vi "Dialog3Stages.vi"(0 "X axis":T2={"Serial port handle"="", "Axis"="", "Controller #"=0, "Min position"=0.0, "Max position"=0.0, "Min velocity"=0.0, "Max velocity"=0.0, "Firmware"="", "Device ID"=0, "Variable event"=refnum, "Variable ref"=refnum, "Resolution, usteps/step"=0, "Serial port semaphore"=refnum, "Joystick buttons"={"MinDir"=1, "MaxDir"=2, "MedSpeed"=5, "HighSpeed"=6}} {"Joystick buttons"."HighSpeed" min=1 max=25 step=1; "Joystick buttons"."MedSpeed" min=1 max=25 step=1; "Joystick buttons"."MaxDir" min=1 max=25 step=1; "Joystick buttons"."MinDir" min=1 max=25 step=1}, 1 "Y axis":T2={"Serial port handle"="", "Axis"="", "Controller #"=0, "Min position"=0.0, "Max position"=0.0, "Min velocity"=0.0, "Max velocity"=0.0, "Firmware"="", "Device ID"=0, "Variable event"=refnum, "Variable ref"=refnum, "Resolution, usteps/step"=0, "Serial port semaphore"=refnum, "Joystick buttons"={"MinDir"=1, "MaxDir"=2, "MedSpeed"=5, "HighSpeed"=6}} {"Joystick buttons"."HighSpeed" min=1 max=25 step=1; "Joystick buttons"."MedSpeed" min=1 max=25 step=1; "Joystick buttons"."MaxDir" min=1 max=25 step=1; "Joystick buttons"."MinDir" min=1 max=25 step=1}, 2 "Z axis":T2={"Serial port handle"="", "Axis"="", "Controller #"=0, "Min position"=0.0, "Max position"=0.0, "Min velocity"=0.0, "Max velocity"=0.0, "Firmware"="", "Device ID"=0, "Variable event"=refnum, "Variable ref"=refnum, "Resolution, usteps/step"=0, "Serial port semaphore"=refnum, "Joystick buttons"={"MinDir"=1, "MaxDir"=2, "MedSpeed"=5, "HighSpeed"=6}} {"Joystick buttons"."HighSpeed" min=1 max=25 step=1; "Joystick buttons"."MedSpeed" min=1 max=25 step=1; "Joystick buttons"."MaxDir" min=1 max=25 step=1; "Joystick buttons"."MinDir" min=1 max=25 step=1}, 3 "Stop event":refnum<user-event>, 4 "Joystick event":T1, 5 "error in":errorcluster={"status"=FALSE, "code"=1073676294, "source"="VISA Read in Zaber TLCM.lvclass:Command.vi:1820008->Zaber TLCM.lvclass:Get home position.vi->Zaber TLCM.lvclass:Get limits.vi->Zaber TLCM.lvclass:Join.vi->Swan probe.vi"}) -> (19 "error out":errorcluster)   [LabVIEW 2018]
uses:
  Zaber.ctl
  GenericDataEvent/GenericEvent.ctl
  ZaberVariables.ctl
  Joystick events/Joystick event.ctl
  <vilib>/Analysis/baseanly.llb/Real Outer Product.vi
  <vilib>/Analysis/NI_AALBase.lvlib
panel:
  in  "ZSlide":dbl(slide)=38.4141345 caption="Z axis, mm" scale format="%#_3f"
  out "XYPositionGraph":dbl[][](graph) caption="XY position graph"
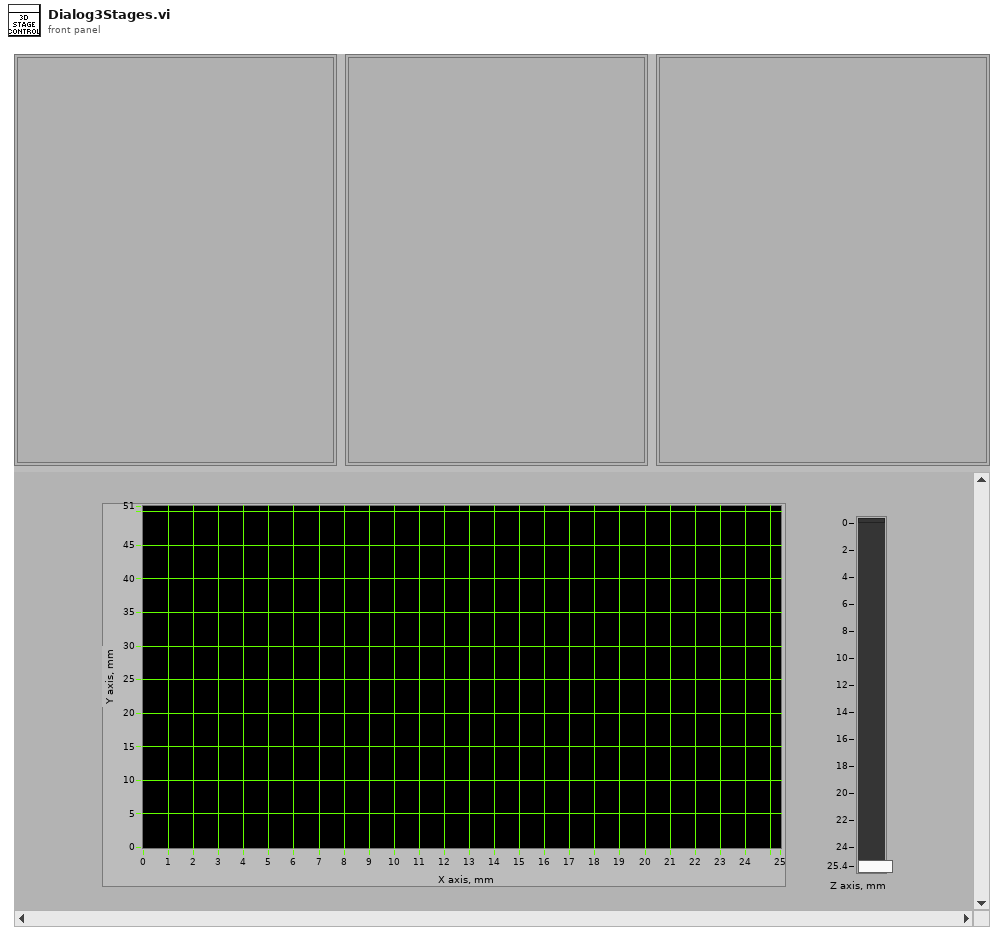
[diagram p1: front panel]
types:
  T1 = typedef "Joystick event.ctl" = refnum<user-event>
  T2 = typedef "Zaber.ctl" = cluster{"Serial port handle":refnum<visa-resource-name>, "Axis":string, "Controller #":u8, "Min position":dbl, "Max position":dbl, "Min velocity":dbl, "Max velocity":dbl, "Firmware":string, "Device ID":i32, "Variable event":T3, "Variable ref":refnum<data-value>, "Resolution, usteps/step":i32, "Serial port semaphore":T4, "Joystick buttons":cluster{"MinDir":i32, "MaxDir":i32, "MedSpeed":i32, "HighSpeed":i32}}
  T3 = typedef "GenericEvent.ctl" = refnum<user-event>
  T4 = typedef "Semaphore RefNum" = refnum<k1>
  T5 = typedef "NI_Matrix.lvlib/RealMatrix.ctl" = dbl[][]
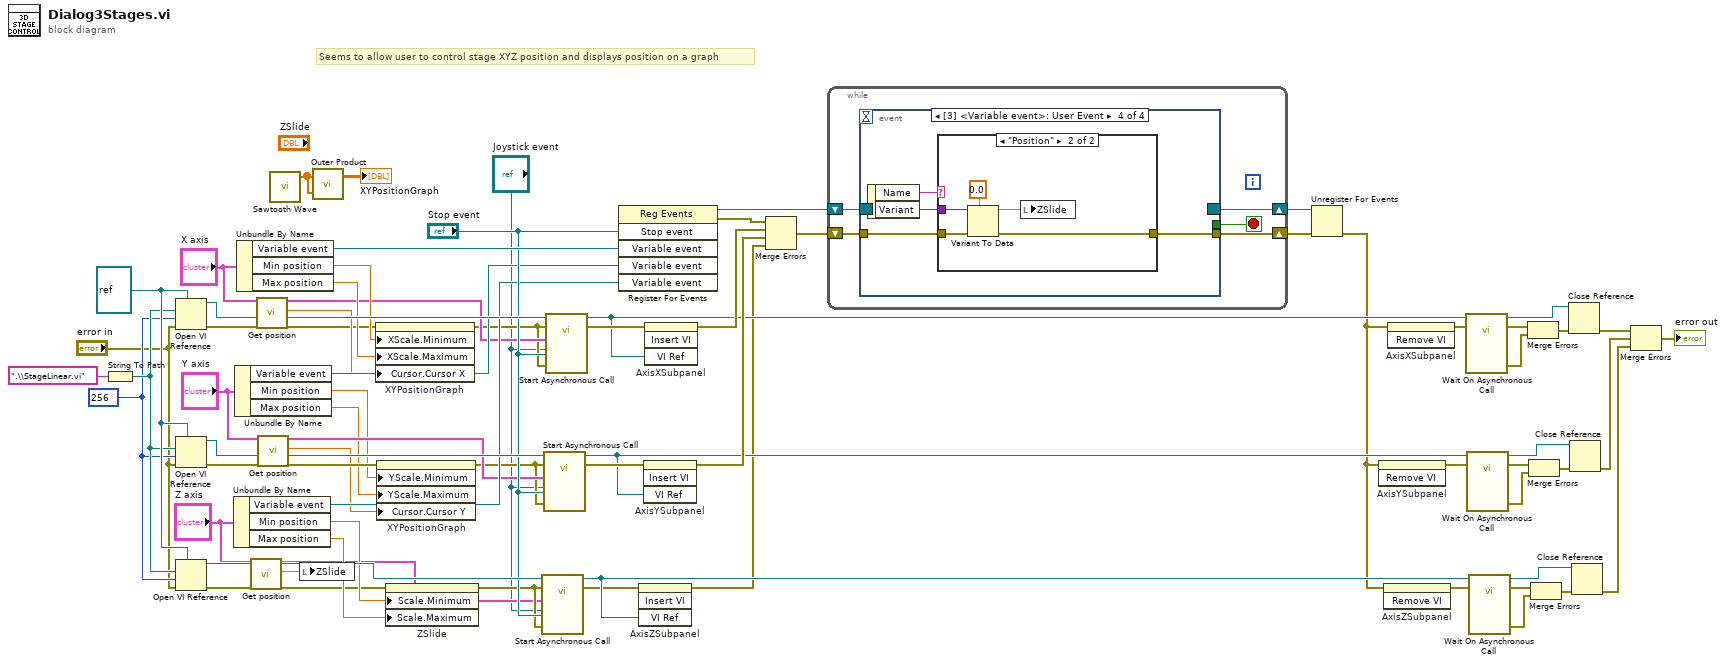
[diagram p0: block diagram]
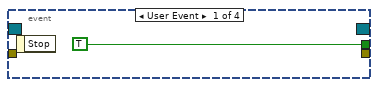
[diagram p2: hidden frame]
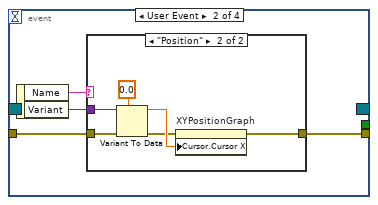
[diagram p3: hidden frame]
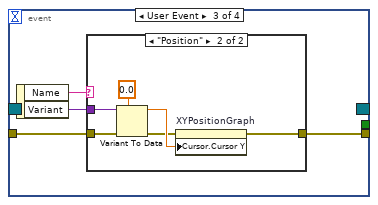
[diagram p5: hidden frame]
diagram:
  w62 = refnum<vi> refnum ("type specifier VI Refnum (for type only)")
  w60 = 256 ("options")
  # "Seems to allow user to control stage XYZ position and displays position on a graph"
  n1 = String To Path(string=".\\StageLinear.vi") -> (path=w61:path)
  n2 = Open VI Reference(type specifier VI Refnum (for type only)=w62, vi path=w61, options=w60, error in (no error)="error in") -> (vi reference=w71:refnum<vi>, error out=w35:errorcluster)  [unwired: 2 in]
  n3 = Open VI Reference(type specifier VI Refnum (for type only)=w62, vi path=w61, options=w60, error in (no error)="error in") -> (vi reference=w64:refnum<vi>, error out=w29:errorcluster)  [unwired: 2 in]
  n4 = Open VI Reference(type specifier VI Refnum (for type only)=w62, vi path=w61, options=w60, error in (no error)="error in") -> (vi reference=w63:refnum<vi>, error out=w18:errorcluster)  [unwired: 2 in]
  n5 = Unbundle By Name("Z axis") -> ("Variable event"=w38:T3, "Min position"=w37:dbl, "Max position"=w36:dbl)
  n6 = Unbundle By Name("Y axis") -> ("Variable event"=w39:T3, "Min position"=w24:dbl, "Max position"=w23:dbl)
  n7 = Unbundle By Name("X axis") -> ("Variable event"=w43:T3, "Min position"=w42:dbl, "Max position"=w41:dbl)
  n8 = call "Get position.vi"("Zaber"="Z axis", "error in"=w18) -> ("Zaber out"=w19:T2, "PositionRb"=w16:dbl, "error out"=w17:errorcluster)  [unwired: 13 in, 2 out]
  n9 = call "Get position.vi"("Zaber"="X axis", "error in"=w35) -> ("Zaber out"=w33:T2, "PositionRb"=w32:dbl, "error out"=w31:errorcluster)  [unwired: 13 in, 2 out]
  n10 = call "Get position.vi"("Zaber"="Y axis", "error in"=w29) -> ("Zaber out"=w27:T2, "PositionRb"=w22:dbl, "error out"=w26:errorcluster)  [unwired: 13 in, 2 out]
  n11 = call <vilib>:"Sawtooth Wave.vi"() -> ("sawtooth wave"=w73:dbl[])  [unwired: 5 in, 2 out]
  n12 = local write "ZSlide"(w16) -> ()
  n13 = call-poly <vilib>:"Outer Product.vi"("Y Vector"=w73, "X Vector"=w73) -> ("Outer Product"=→"XYPositionGraph":T5)  [unwired: 1 out]
  n14 = property on="XYPositionGraph" class="IntGraph (strict)"(error in=w31, "XScale.Minimum"=w42, "XScale.Maximum"=w41, "Cursor.Cursor X"=w32) -> (error out=w30:errorcluster)  [unwired: 1 in, 1 out]
  n15 = property on="XYPositionGraph" class="IntGraph (strict)"(error in=w26, "YScale.Minimum"=w24, "YScale.Maximum"=w23, "Cursor.Cursor Y"=w22) -> (error out=w25:errorcluster)  [unwired: 1 in, 1 out]
  n16 = property on="ZSlide" class="Slide (strict)"(error in=w17, "Scale.Minimum"=w37, "Scale.Maximum"=w36) -> (error out=w21:errorcluster)  [unwired: 1 in, 1 out]
  n17 = call-by-ref "Start Asynchronous Call"(reference=w63, error in=w21, "Axis"=w19, "Joystick event"="Joystick event", "Stop event"="Stop event", "error in"=w21) -> (reference out=w7:refnum<vi>, error out=w6:errorcluster)  [unwired: 14 in, 2 out]
  n18 = call-by-ref "Start Asynchronous Call"(reference=w64, error in=w25, "Axis"=w27, "Joystick event"="Joystick event", "Stop event"="Stop event", "error in"=w25) -> (reference out=w13:refnum<vi>, error out=w15:errorcluster)  [unwired: 14 in, 2 out]
  n19 = call-by-ref "Start Asynchronous Call"(reference=w71, error in=w30, "Axis"=w33, "Joystick event"="Joystick event", "Stop event"="Stop event", "error in"=w30) -> (reference out=w9:refnum<vi>, error out=w11:errorcluster)  [unwired: 14 in, 2 out]
  n20 = register-events("Stop event", w43, w39, w38) -> (reference out=w66:refnum<event-registration>, error out=w65:errorcluster)  [unwired: 2 in]
  n21 = invoke on="AxisZSubpanel" class="SubPnl" method="Insert VI"(error in=w6, "VI Ref"=w7) -> (error out=w5:errorcluster)  [unwired: 2 in, 3 out]
  n22 = invoke on="AxisYSubpanel" class="SubPanel" method="Insert VI"(error in=w15, "VI Ref"=w13) -> (error out=w14:errorcluster)  [unwired: 2 in, 3 out]
  n23 = invoke on="AxisXSubpanel" class="SubPnl" method="Insert VI"(error in=w11, "VI Ref"=w9) -> (error out=w10:errorcluster)  [unwired: 2 in, 3 out]
  n24 = Merge Errors(w65, w10, w14, w5) -> (w59:errorcluster)
  n25 = while {
    shift-right: [w76] -> w57
    shift-left: w66 -> [w78]
    shift-right: [w74] -> w58
    shift-left: w59 -> [w75]
    stop <- w77 stop-if-true
    n26 = event shown="[3] <Variable event>: User Event" {
      selector: w78 -> [_ _ _ _]
      dyn-events: [_ _ _ _] -> w76
      timeout: _ -> [_ _ _ _]
      tunnel: [TRUE _ _ _] -> w77
      tunnel: w75 -> [_ w81 w92 w103]
      tunnel: [_ w80 w91 w102] -> w74
      event User Event {
        n27 = event-data() -> ()  [unwired: 1 in, 1 out]
      }
      event User Event {
        n28 = event-data() -> ("Name"=w83:string, "Variant"=w82:variant)  [unwired: 1 in]
        n29 = case shown="\"Position\"" w83 {
          tunnel: w82 -> [_ w90]
          tunnel: w81 -> [w84 w87]
          tunnel: [w84 w85] -> w80
          frame Default {
          }
          frame "Position" {
            n30 = Variant To Data(error in=w87, type=0.0, Variant=w90) -> (data=w89:dbl, error out=w86:errorcluster)
            n31 = property on="XYPositionGraph" class="IntGraph (strict)"(error in=w86, "Cursor.Cursor X"=w89) -> (error out=w85:errorcluster)  [unwired: 1 in, 1 out]
          }
        }
      }
      event User Event {
        n32 = event-data() -> ("Name"=w94:string, "Variant"=w93:variant)  [unwired: 1 in]
        n33 = case shown="\"Position\"" w94 {
          tunnel: w93 -> [_ w101]
          tunnel: w92 -> [w95 w98]
          tunnel: [w95 w96] -> w91
          frame Default {
          }
          frame "Position" {
            n34 = Variant To Data(error in=w98, type=0.0, Variant=w101) -> (data=w100:dbl, error out=w97:errorcluster)
            n35 = property on="XYPositionGraph" class="IntGraph (strict)"(error in=w97, "Cursor.Cursor Y"=w100) -> (error out=w96:errorcluster)  [unwired: 1 in, 1 out]
          }
        }
      }
      event User Event {
        n36 = event-data() -> ("Name"=w105:string, "Variant"=w104:variant)  [unwired: 1 in]
        n37 = case shown="\"Position\"" w105 {
          tunnel: w104 -> [_ w111]
          tunnel: w103 -> [w106 w109]
          tunnel: [w106 w108] -> w102
          frame Default {
          }
          frame "Position" {
            n38 = Variant To Data(error in=w109, type=0.0, Variant=w111) -> (data=w107:dbl, error out=w108:errorcluster)
            n39 = local write "ZSlide"(w107) -> ()
          }
        }
      }
    }
  }
  n40 = Unregister For Events(event registration refnum=w57, error in=w58) -> (error out=w4:errorcluster)
  n41 = invoke on="AxisYSubpanel" class="SubPanel" method="Remove VI"(error in=w4) -> (error out=w12:errorcluster)  [unwired: 2 in, 2 out]
  n42 = invoke on="AxisZSubpanel" class="SubPnl" method="Remove VI"(error in=w4) -> (error out=w3:errorcluster)  [unwired: 2 in, 2 out]
  n43 = invoke on="AxisXSubpanel" class="SubPnl" method="Remove VI"(error in=w4) -> (error out=w8:errorcluster)  [unwired: 2 in, 2 out]
  n44 = call-by-ref "Wait On Asynchronous Call"(reference=w9, error in=w8) -> (reference out=w67:refnum<vi>, error out=w69:errorcluster, 19:"error out"=w56:errorcluster)  [unwired: 18 in, 1 out]
  n45 = call-by-ref "Wait On Asynchronous Call"(reference=w13, error in=w12) -> (reference out=w53:refnum<vi>, error out=w55:errorcluster, 19:"error out"=w52:errorcluster)  [unwired: 18 in, 1 out]
  n46 = call-by-ref "Wait On Asynchronous Call"(reference=w7, error in=w3) -> (reference out=w49:refnum<vi>, error out=w51:errorcluster, 19:"error out"=w48:errorcluster)  [unwired: 18 in, 1 out]
  n47 = Merge Errors(w69, w56) -> (w68:errorcluster)
  n48 = Merge Errors(w55, w52) -> (w54:errorcluster)
  n49 = Merge Errors(w51, w48) -> (w50:errorcluster)
  n50 = Close Reference(reference=w67, error in (no error)=w68) -> (error out=w47:errorcluster)
  n51 = Close Reference(reference=w53, error in (no error)=w54) -> (error out=w46:errorcluster)
  n52 = Close Reference(reference=w49, error in (no error)=w50) -> (error out=w45:errorcluster)
  n53 = Merge Errors(w47, w46, w45) -> (→"error out":errorcluster)
